vi "FIR Filter with I.C. (CDB).vi"(6 "Initial X Conditions":cdb[](array[numeric]), 7 "FIR Coefficients":dbl[](array[numeric]), 10 "X":cdb[](array[numeric])) -> (0 "Final X Conditions":cdb[](array[numeric]), 2 "error":i32, 3 "Filtered X":cdb[](array[numeric]))   [LabVIEW 2017, in "NI_AALBase.lvlib"]
doc: "Filters the input sequence <B>X</B> using the direct-form FIR filter specified by <B>FIR Coefficients</B>. You can use this VI to process blocks of continuous data. Wire data to the <B>X</B> input to determine the polymorphic instance to use or manually select the instance."
uses:
  NI_AALBase.lvlib
  lvanlys.dll
panel:
  # "FIR Filter with I.C."
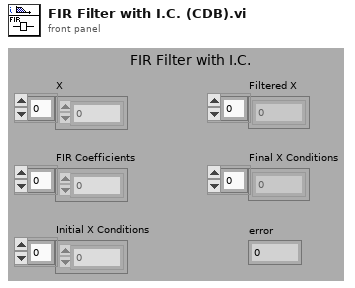
[diagram p1: front panel]
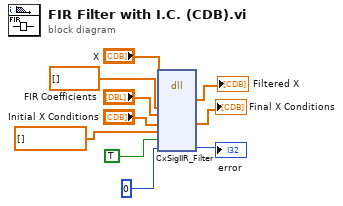
[diagram p0: block diagram]
diagram:
  n1 = dll-call lib="C:/Program Files/National Instruments/LabVIEW 2017/resource/lvanlys.*" fn="CxSigIIR_Filter"("X"="X", "aH"=dbl[] [] ("Reverse Coefficients"), "bH"="FIR Coefficients", "Initial X Conditions"="Initial X Conditions", "X"=cdb[] [], "output param"=TRUE, "dsperr"=0) -> ("X"=→"Filtered X":cdb[], "Initial X Conditions"=→"Final X Conditions":cdb[], "dsperr"=→"error":i32)  [unwired: 8 in, 2 out]
